vi "Direction Safety.vi"(1 "Min Rate":dbl, 2 "Desired Rate":dbl, 3 "Encoder Rate":dbl) -> (0 "Super Safe Rate":dbl)   [LabVIEW 2013]
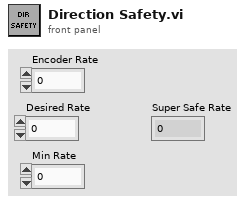
[diagram p1: front panel]
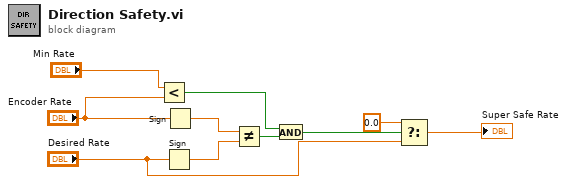
[diagram p0: block diagram]
diagram:
  n1 = Less?(x="Min Rate", y="Encoder Rate") -> (x < y?=w2:bool)
  n2 = Sign(1:"Desired Rate") -> (0:w7:dbl)
  n3 = Sign(1:"Encoder Rate") -> (0:w8:dbl)
  n4 = Not Equal?(x=w8, y=w7) -> (x != y?=w3:bool)
  n5 = And(x=w2, y=w3) -> (x .and. y?=w1:bool)
  n6 = Select(t=0.0, s=w1, f="Desired Rate") -> (s? t:f=→"Super Safe Rate":dbl)
